vi "test highlight.vi"() -> ()   [LabVIEW 2017]
uses:
  <vilib>/Utility/traverseref.llb/TRef TravTarget.ctl
  <vilib>/Utility/traverseref.llb/VI Scripting - Traverse.lvlib
panel:
  in  "Value":string="Data: Initialize\nInitialize Core Data\nData: Load DataCache\nEvents: Register\nUI: Front Panel State >> Open //Open | Close\nUI: Initialize\n\n//Register\nError Occurred@* >> Error Handler -><register> //comments\nSystemlink Connected@SystemlinkClient >> Action: Record Status Change -><register>\nSystemlink Disconnected@SystemlinkClient >> Action: Record Status Change -><register> //comments\n//Full Minute Trigger@Scheduler >> Macro: Update UI -><register>\nFull Hour Trigger@Scheduler >> Macro: Scheduled Task -><register>\n\n//Send Messages to Client\nData: Set Configuration >> Server.Address:${Systemlink.Server:127.0.0.1:8000} ->| SystemlinkClient\nData: Set Configuration >> Server.UserName:${Systemlink.Username} -> SystemlinkClient\nData: Set Configuration >> Server.Passwords:${Systemlink.passwords} -> SystemlinkClient\nSystemlink: Connect to Server -> SystemlinkClient //comments\n\n//Send Messages to Scheduler\nAPI: Enable Full Minute Trigger >> On -@ Scheduler\nAPI: Enable Full Hour Trigger >> off -@ Scheduler\n\n//unregister\nError Occurred@* >> Error Handler -><unregister> \nSystemlink Connected@SystemlinkClient >> Action: Record Status Change -><unregister>\nSystemlink Disconnected@SystemlinkClient >> Action: Record Status Change -><unregister>\n\n"
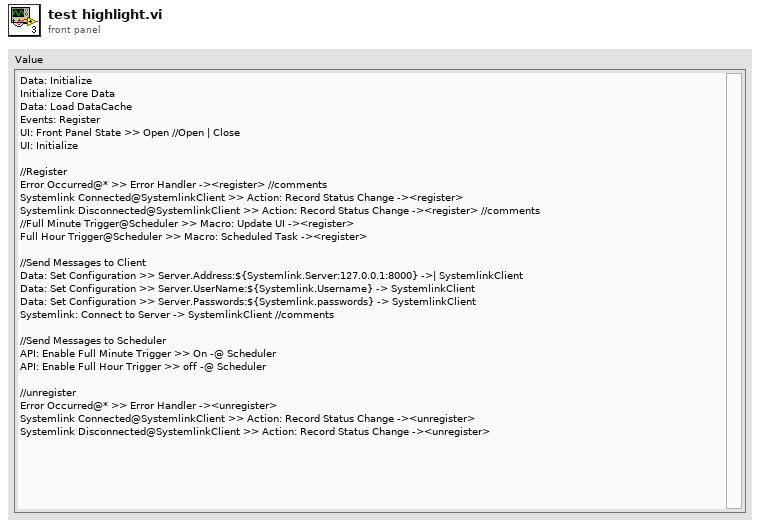
[diagram p1: front panel]
types:
  T1 = typedef "TRef TravTarget.ctl" = enum16{"FP", "BD", "Other"}
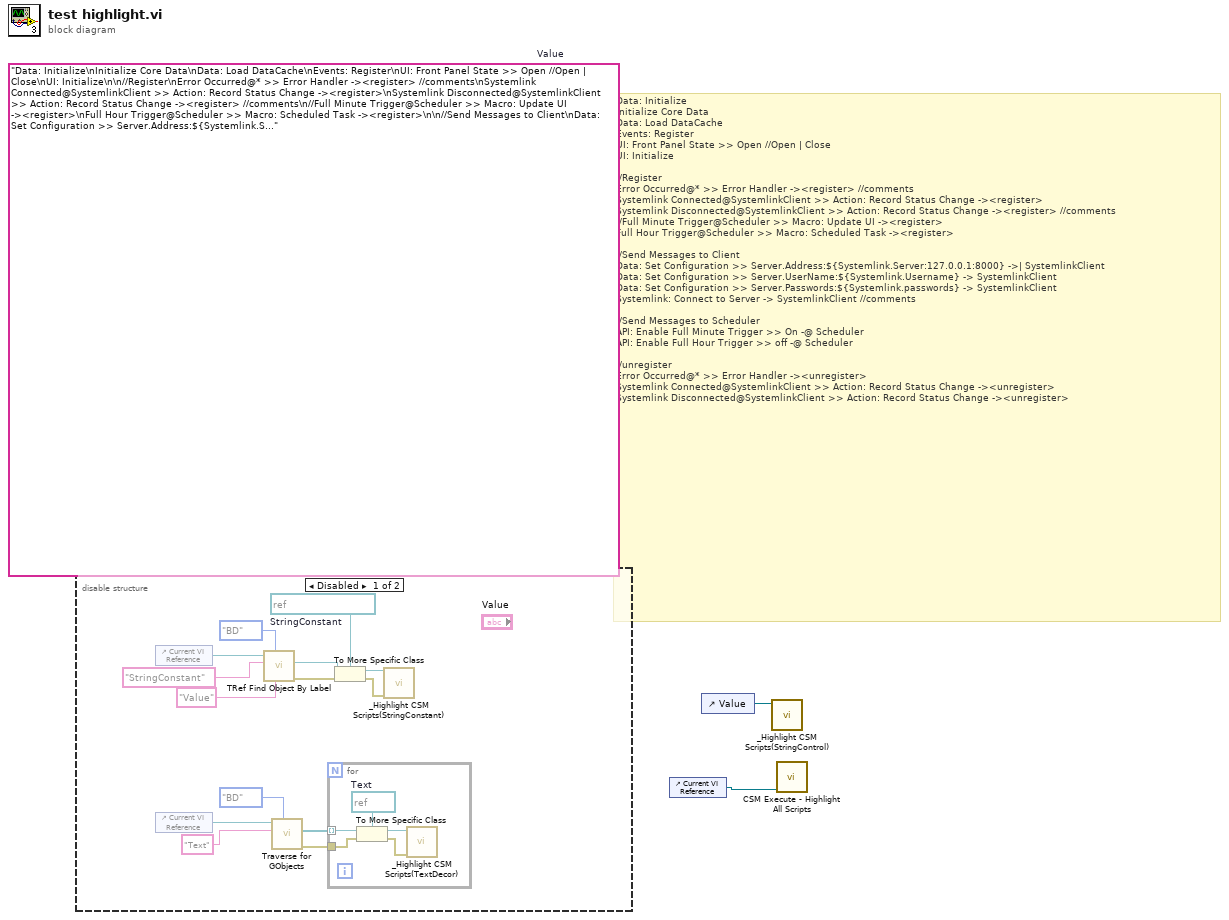
[diagram p0: block diagram]
diagram:
  (unwired) "Data: Initialize\nInitialize Core Data\nData: Load DataCache\nEvents: Register\nUI: Front Panel State >> Open //Open | Close\nUI: Initialize\n\n//Register\nError Occurred@* >> Error Handler -><register> //comments\nSystemlink Connected@SystemlinkClient >> Action: Record Status Change -><register>\nSystemlink Disconnected@SystemlinkClient >> Action: Record Status Change -><register> //comments\n//Full Minute Trigger@Scheduler >> Macro: Update UI -><register>\nFull Hour Trigger@Scheduler >> Macro: Scheduled Task -><register>\n\n//Send Messages to Client\nData: Set Configuration >> Server.Address:${Systemlink.Server:127.0.0.1:8000} ->| SystemlinkClient\nData: Set Configuration >> Server.UserName:${Systemlink.Username} -> SystemlinkClient\nData: Set Configuration >> Server.Passwords:${Systemlink.passwords} -> SystemlinkClient\nSystemlink: Connect to Server -> SystemlinkClient //comments\n\n//Send Messages to Scheduler\nAPI: Enable Full Minute Trigger >> On -@ Scheduler\nAPI: Enable Full Hour Trigger >> off -@ Scheduler\n\n//unregister\nError Occurred@* >> Error Handler -><unregister> \nSystemlink Connected@SystemlinkClient >> Action: Record Status Change -><unregister>\nSystemlink Disconnected@SystemlinkClient >> Action: Record Status Change -><unregister>\n\n"  # Value
  # "Data: Initialize\nInitialize Core Data\nData: Load DataCache\nEvents: Register\nUI: Front Panel State >> Open //Open | Close\nUI: Initialize\n\n//Register\nError Occurred@* >> Error Handler -><register> //comments\nSystemlink Connected@SystemlinkClient >> Action: Record Status Change -><register>\nSystemlink Disconnected@SystemlinkClient >> Action: Record Status Change -><register> //comments\n//Full Minute Trigger@Scheduler >> Macro: Update UI -><register>\nFull Hour Trigger@Scheduler >> Macro: Scheduled Task -><register>\n\n//Send Messages to Client\nData: Set Configuration >> Server.Address:${Systemlink.Server:127.0.0.1:8000} ->| SystemlinkClient\nData: Set Configuration >> Server.UserName:${Systemlink.Username} -> SystemlinkClient\nData: Set Configuration >> Server.Passwords:${Systemlink.passwords} -> SystemlinkClient\nSystemlink: Connect to Server -> SystemlinkClient //comments\n\n//Send Messages to Scheduler\nAPI: Enable Full Minute Trigger >> On -@ Scheduler\nAPI: Enable Full Hour Trigger >> off -@ Scheduler\n\n//unregister\nError Occurred@* >> Error Handler -><unregister> \nSystemlink Connected@SystemlinkClient >> Action: Record Status Change -><unregister>\nSystemlink Disconnected@SystemlinkClient >> Action: Record Status Change -><unregister>"
  n1 = disable-structure shown="Disabled" {
    frame Disabled {
      w11 = refnum<vi> refnum  # StringConstant
      n2 = control-ref of="Current VI Reference"() -> (w16:refnum<vi>)
      n3 = control-ref of="Current VI Reference"() -> (w6:refnum<vi>)
      n4 = call <vilib>:"TRef Find Object By Label.vi"("Label"="Value", "Traverse Target"=TRef_TravTarget."BD", "Class Name"="StringConstant", "VI Ref"=w16) -> ("error out"=w13:errorcluster, "Found Obj Ref"=w12:refnum<vi>)  [unwired: 4 in, 2 out]
      n5 = call <vilib>:"Traverse for GObjects.vi"("Traverse Target"=TRef_TravTarget."BD", "Class Name"="Text", "VI Refnum"=w6) -> ("error out"=w3:errorcluster, "References"=w4:refnum<vi>[])  [unwired: 5 in, 2 out]
      n6 = for {
        tunnel: w4 -> [w18] mode=indexing
        tunnel: w3 -> [w17]
        w21 = refnum<vi> refnum  # Text
        n7 = To More Specific Class(target class=w21, reference=w18, error in=w17) -> (specific class reference=w20:refnum<vi>, error out=w19:errorcluster)
        n8 = call "_Highlight CSM Scripts(TextDecor).vi"("error in (no error)"=w19, "reference out 2"=w20) -> ()  [unwired: 9 in, 1 out]
      }
      n9 = To More Specific Class(target class=w11, reference=w12, error in=w13) -> (specific class reference=w10:refnum<vi>, error out=w9:errorcluster)
      n10 = call "_Highlight CSM Scripts(StringConstant).vi"("error in (no error)"=w9, "reference out"=w10) -> ()  [unwired: 9 in, 1 out]
    }
    frame Enabled {
    }
  }
  n11 = control-ref of="Current VI Reference"() -> (w2:refnum<vi>)
  n12 = control-ref of="Value"() -> (w1:refnum<vi>)
  n13 = call "_Highlight CSM Scripts(StringControl).vi"("String Ctrl"=w1) -> ()  [unwired: 11 in]
  n14 = call "CSM Execute - Highlight All Scripts.vi"("User VI Ref"=w2) -> ()  [unwired: 10 in, 1 out]
